vi "Restore Configuration.vi"(8 "error in (no error)":errorcluster, 10 "File path":path, 11 "Measure Object in":refnum<class "Measure Object.lvclass">) -> (0 "error out":errorcluster, 1 "Section out":string, 2 "File path out":path, 3 "Measure Object out":refnum<class "Measure Object.lvclass">)   [LabVIEW 2015, in "Measure Object.lvclass"]
uses:
  Measure Object.lvclass
  Measure Object.lvclass/Measure Object.ctl
  Measure Object Messages/Restore Configuration Msg/Restore Configuration Msg.lvclass/Restore Configuration Msg.ctl
  <vilib>/ActorFramework/Message Enqueuer/Message Enqueuer.lvclass/Message Enqueuer.ctl
  Read Name.vi
  <vilib>/ActorFramework/Message Enqueuer/Enqueue.vi
  <vilib>/ActorFramework/Message Priority Queue/Priority Enqueue.vi
  Measure Object Messages/Restore Configuration Msg/Restore Configuration Msg.lvclass
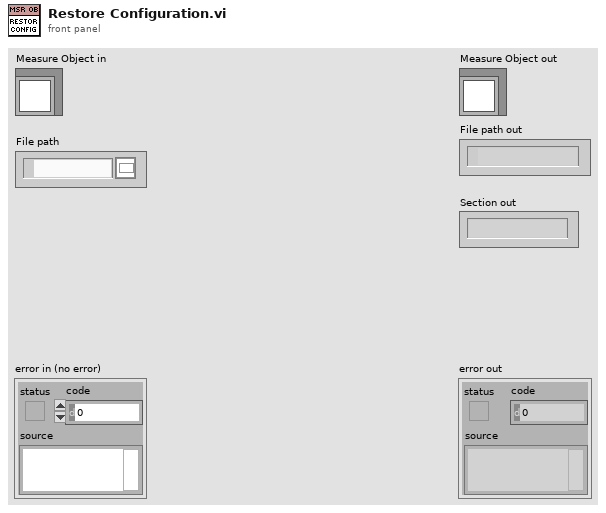
[diagram p1: front panel]
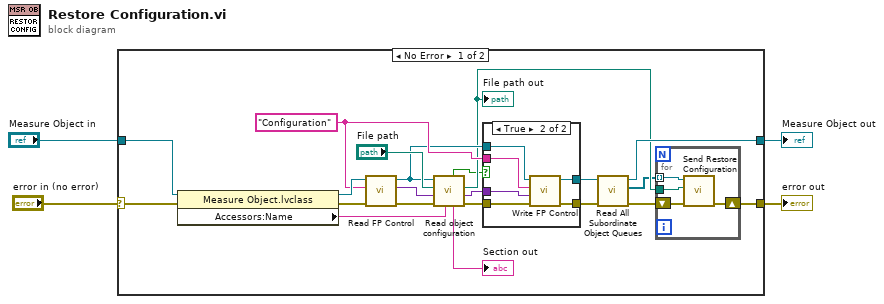
[diagram p0: block diagram]
diagram:
  n1 = case shown="No Error" "error in (no error)" {
    selector: "error in (no error)" -> [w21 w39]
    tunnel: [w7 w39] -> w3
    tunnel: [w11 w38] -> w1
    tunnel: "Measure Object in" -> [w20 w38]
    frame No Error {
      w17 = "Configuration" ("Control Name")
      n2 = property class="Measure Object.lvclass"(reference=w20, error in=w21) -> (reference out=w19:refnum<class "Measure Object.lvclass">, error out=w22:errorcluster, "Accessors:Name"=w18:string)
      n3 = call-dynamic "Read FP Control.vi"("error in (no error)"=w22, "Control Name"=w17, "Measure Object in"=w19) -> ("error out"=w23:errorcluster, "Control Value"=w25:variant, "Measure Object out"=w14:refnum<class "Measure Object.lvclass">)  [unwired: 5 in, 1 out]
      n4 = call "Read object configuration.vi"("Object name"=w18, "Error In"=w23, "type"=w25, "File path"="File path", "object"=w14) -> ("Error Out"=w15:errorcluster, "Configuration"=w16:variant, "File path out"=w10:path, "Section out"=→"Section out":string, "found?"=w5:bool)  [unwired: 2 in]
      "File path out" <- w10
      n5 = case shown="True" w5 {
        tunnel: w17 -> [_ w33]
        tunnel: w16 -> [_ w32]
        tunnel: w15 -> [w27 w31]
        tunnel: w14 -> [w26 w30]
        tunnel: [w27 w29] -> w13
        tunnel: [w26 w28] -> w12
        frame False {
        }
        frame True {
          n6 = call-dynamic "Write FP Control.vi"("error in (no error)"=w31, "Control Value"=w32, "Control Name"=w33, "Measure Object in"=w30) -> ("error out"=w29:errorcluster, "Measure Object out"=w28:refnum<class "Measure Object.lvclass">)  [unwired: 6 in]
        }
      }
      n7 = call-dynamic "Read All Subordinate Object Queues.vi"("error in (no error)"=w13, "Measure Object in"=w12) -> ("error out"=w8:errorcluster, "Object enqueuers"=w9:refnum<class "Message Enqueuer.lvclass">[], "Measure Object out"=w11:refnum<class "Measure Object.lvclass">)  [unwired: 6 in, 1 out]
      n8 = for {
        tunnel: w10 -> [w37]
        tunnel: w9 -> [w36] mode=indexing
        shift-right: [w35] -> w7
        shift-left: w8 -> [w34]
        n9 = call "Send Restore Configuration.vi"("error in (no error)"=w34, "File path"=w37, "Message Enqueuer"=w36) -> ("error out"=w35:errorcluster)  [unwired: 7 in, 1 out]
      }
    }
    frame Error {
    }
  }
  "error out" <- w3
  "Measure Object out" <- w1
